vi "Generate INSERT Query for Transaction Table.vi"(8 "error in (no error)":errorcluster, 11 "Statement in":refnum<class "TransactionList.lvclass">) -> (0 "error out":errorcluster, 2 "Insert Query":string, 3 "Statement out":refnum<class "TransactionList.lvclass">)   [LabVIEW 2018, in "TransactionList.lvclass"]
uses:
  TransactionList.lvclass
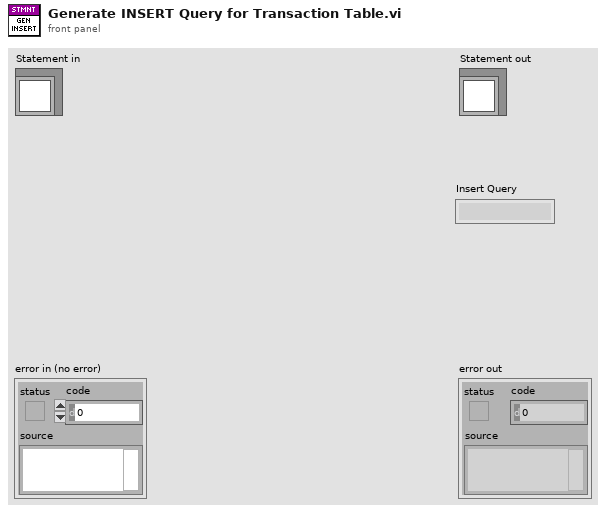
[diagram p1: front panel]
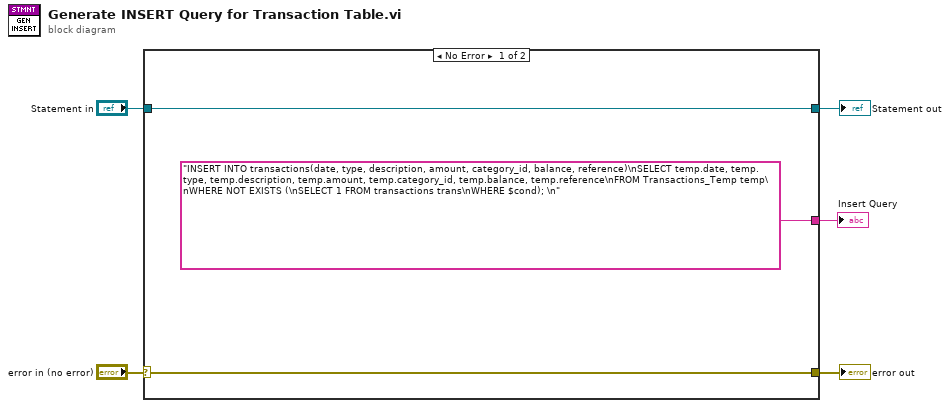
[diagram p0: block diagram]
diagram:
  n1 = case shown="No Error" "error in (no error)" {
    selector: "error in (no error)" -> [w7 w10]
    tunnel: [w7 w10] -> w4
    tunnel: [w8 w9] -> w2
    tunnel: "Statement in" -> [w8 w9]
    tunnel: ["INSERT INTO transactions(date, type, description, amount, category_id, balance, reference)\nSELECT temp.date, temp.type, temp.description, temp.amount, temp.category_id, temp.balance, temp.reference\nFROM Transactions_Temp temp\nWHERE NOT EXISTS (\nSELECT 1 FROM transactions trans\nWHERE $cond); \n" _] -> w1
    frame No Error {
    }
    frame Error {
    }
  }
  "error out" <- w4
  "Statement out" <- w2
  "Insert Query" <- w1
